vi "Stimulus-Initialize (V3).vi"(0 "Stimulus Channel":T1={"Waveform"={"Type"=enum."OFF", "Tone"={"Frequency (kHz)"=0.0, "Last Freq"=0.0, "Last Phase"=0.0}, "Pulse Train"={"Pulse width (us)"=0.0, "Pulse rate (Hz)"=0.0, "Gap (ms)"=0.0, "Polarity"=enum."POS", "PT State"={"Template"=[], "Nperiod"=0, "Index"=0, "Pulse Rate (Hz)"=0.0, "Phase (cycles)"=0.0, "Noff"=0}, "Asynch"=FALSE}, "Noise"={"InvFilt"=FALSE, "Noise"=[], "CurPt"=0, "Aweight"=FALSE, "Seed"=0, "afile"=path ""}, "File"={"Filename"=path "", "Signal"=[], "Channel"=0, "stream"=FALSE, "offset"=0, "nreps"=0, "loops"=0}, "FMSweep"={"Rate (oct/s)"=0.0, "Fmin (Hz)"=0.0, "Fmax (Hz)"=0.0, "Ramp (ms)"=0.0, "Linear"=FALSE}, "Chirp Train"={"Params"={"Fmin (kHz)"=4.0, "Fmax (kHz)"=64.0, "Compensate"=FALSE, "Duration (ms)"=2.0}, "Data"={"WF"=[]}}, "Complex Tone"={"Params"={"F0 (Hz)"=0.0, "Band"={"Flow (Hz)"=0.0, "Fhigh (Hz)"=0.0}, "Phase"=enum."Cosine", "Min F0 (Hz)"=0.0, "Max F0 (Hz)"=0.0, "ContinRandPhase"=FALSE, "Max peak factor"=inf, "Max mod depth"=2.0, "MinHarmNum"=0, "MaxHarmNum"=0, "Level Mode"=enum."per component", "% jitter"=0.0}, "Data"={"Ncomp"=0, "MinHarm"=0, "Phase"=[], "Amplitude"=[], "Npts/frame"=0, "Last F0"=0.0, "Fmin"=0.0, "Fmax"=0.0, "Lslope"=0.0, "randphase"=FALSE, "overall rms"=FALSE, "fmult"=[], "jittered"=FALSE}}, "Moving Ripple"={"Params"={"Fmin"=0.0, "Fmax"=0.0, "Density"=0.0, "Velocity"=0.0, "Depth"=0.0, "Phase"=0.0, "Comp/oct"=0}, "Data"={"Freq"=[], "A"=[], "phase"=[], "Phase"=0.0}}}, "Filter"={"Type"=enum."Lowpass", "CF (kHz)"=0.0, "BW (kHz)"=0.0, "Cascade"=FALSE, "Quadrature"=FALSE, "Scale Factor"=0.0, "Stages"=[], "Class"=enum."Elliptic", "Order"=0, "BWUnits"=enum."Linear"}, "Burst"={"Active"=FALSE, "Delay (ms)"=0.0, "Duration (ms)"=0.0, "Ramp (ms)"=0.0, "Rate (Hz)"=0.0, "Trepeat (ms)"=0.0, "Repeat"=FALSE}, "Level"={"Level"=0.0, "Units"=enum."dB atten", "Max"=0.0, "Multiplier"=0.0, "Cal File"=path "", "Cal"={"Freq (Hz)"=[], "Mag (dB SPL)"=[], "Phase (deg)"=[]}}, "Name"="", "Advanced"={"Rep Mask"="", "AltPol"=FALSE, "Var"="", "Expr"="", "Persist"=FALSE}, "SAM"={"Active"=FALSE, "Frequency (Hz)"=0.0, "Depth"=0.0, "Init Phase (cycles)"=0.0, "phase (degrees)"=0.0, "Asynch"=FALSE}, "Destination"={"Name"="", "Num"=0}} {"Filter"."Stages"."IIR Filter"."Forward Coefficients" format="%.4f"; "Filter"."Stages"."IIR Filter"."Reverse Coefficients" format="%.4f"}, 7 "Sampling rate (Hz)":dbl, 9 "Npts":i32, 11 "error in (no error)":errorcluster) -> (4 "Stimulus Channel out":T1={"Waveform"={"Type"=enum."OFF", "Tone"={"Frequency (kHz)"=0.0, "Last Freq"=0.0, "Last Phase"=0.0}, "Pulse Train"={"Pulse width (us)"=0.0, "Pulse rate (Hz)"=0.0, "Gap (ms)"=0.0, "Polarity"=enum."POS", "PT State"={"Template"=[], "Nperiod"=0, "Index"=0, "Pulse Rate (Hz)"=0.0, "Phase (cycles)"=0.0, "Noff"=0}, "Asynch"=FALSE}, "Noise"={"InvFilt"=FALSE, "Noise"=[], "CurPt"=0, "Aweight"=FALSE, "Seed"=0, "afile"=path ""}, "File"={"Filename"=path "", "Signal"=[], "Channel"=0, "stream"=FALSE, "offset"=0, "nreps"=0, "loops"=0}, "FMSweep"={"Rate (oct/s)"=0.0, "Fmin (Hz)"=0.0, "Fmax (Hz)"=0.0, "Ramp (ms)"=0.0, "Linear"=FALSE}, "Chirp Train"={"Params"={"Fmin (kHz)"=4.0, "Fmax (kHz)"=64.0, "Compensate"=FALSE, "Duration (ms)"=2.0}, "Data"={"WF"=[]}}, "Complex Tone"={"Params"={"F0 (Hz)"=0.0, "Band"={"Flow (Hz)"=0.0, "Fhigh (Hz)"=0.0}, "Phase"=enum."Cosine", "Min F0 (Hz)"=0.0, "Max F0 (Hz)"=0.0, "ContinRandPhase"=FALSE, "Max peak factor"=inf, "Max mod depth"=2.0, "MinHarmNum"=0, "MaxHarmNum"=0, "Level Mode"=enum."per component", "% jitter"=0.0}, "Data"={"Ncomp"=0, "MinHarm"=0, "Phase"=[], "Amplitude"=[], "Npts/frame"=0, "Last F0"=0.0, "Fmin"=0.0, "Fmax"=0.0, "Lslope"=0.0, "randphase"=FALSE, "overall rms"=FALSE, "fmult"=[], "jittered"=FALSE}}, "Moving Ripple"={"Params"={"Fmin"=0.0, "Fmax"=0.0, "Density"=0.0, "Velocity"=0.0, "Depth"=0.0, "Phase"=0.0, "Comp/oct"=0}, "Data"={"Freq"=[], "A"=[], "phase"=[], "Phase"=0.0}}}, "Filter"={"Type"=enum."Lowpass", "CF (kHz)"=0.0, "BW (kHz)"=0.0, "Cascade"=FALSE, "Quadrature"=FALSE, "Scale Factor"=0.0, "Stages"=[], "Class"=enum."Elliptic", "Order"=0, "BWUnits"=enum."Linear"}, "Burst"={"Active"=FALSE, "Delay (ms)"=0.0, "Duration (ms)"=0.0, "Ramp (ms)"=0.0, "Rate (Hz)"=0.0, "Trepeat (ms)"=0.0, "Repeat"=FALSE}, "Level"={"Level"=0.0, "Units"=enum."dB atten", "Max"=0.0, "Multiplier"=0.0, "Cal File"=path "", "Cal"={"Freq (Hz)"=[], "Mag (dB SPL)"=[], "Phase (deg)"=[]}}, "Name"="", "Advanced"={"Rep Mask"="", "AltPol"=FALSE, "Var"="", "Expr"="", "Persist"=FALSE}, "SAM"={"Active"=FALSE, "Frequency (Hz)"=0.0, "Depth"=0.0, "Init Phase (cycles)"=0.0, "phase (degrees)"=0.0, "Asynch"=FALSE}, "Destination"={"Name"="", "Num"=0}} {"Filter"."Stages"."IIR Filter"."Forward Coefficients" format="%.4f"; "Filter"."Stages"."IIR Filter"."Reverse Coefficients" format="%.4f"}, 6 "Max Level":dbl, 15 "error out":errorcluster)   [LabVIEW 2015]
uses:
  Controls/Advanced Filter XCtl/Filter Data.ctl
  Controls/Advanced Filter XCtl/Advanced Filter XCtl.xctl
  Controls/Level XCtl/Level Units.ctl
  Controls/Level XCtl/Level Data.ctl
  Controls/Level XCtl/Level XCtl.xctl
  Controls/Burst XCtl/Burst Data.ctl
  Controls/Burst XCtl/Burst Control.xctl
  Controls/Waveform XCtl/Waveform Enum.ctl
  Waveform VIs/Tone VIs/Tone Params.ctl
  Waveform VIs/Pulse Train VIs/Pulse Polarity.ctl
  Waveform VIs/Pulse Train VIs/PT-Continuous State.ctl
  Waveform VIs/Pulse Train VIs/Pulse Train Params.ctl
  Waveform VIs/Noise VIs/Noise Params.ctl
  Waveform VIs/File VIs/StimFile-Params.ctl
  Waveform VIs/FM Sweep VIs/FM Sweep Params.ctl
  Controls/Waveform XCtl/Waveform Data.ctl
  Controls/Waveform XCtl/Waveform XCtl.xctl
  Controls/Advanced Options XCtl/Advanced Stimulus Options.ctl
  Controls/Advanced Options XCtl/Advanced Stimulus Options.xctl
  Modulation VIs/SAM VIs/SAM Params.ctl
  Waveform VIs/Chirp Train VIs/Chirp Train Params.ctl
  Waveform VIs/Chirp Train VIs/Chirp Train.ctl
  Waveform VIs/Complex Tone VIs/CT-Phase Enum.ctl
  Waveform VIs/Complex Tone VIs/CT-Params.ctl
  Waveform VIs/Complex Tone VIs/CT-Runtime Data.ctl
  Filter VIs/Filter-Bandwidth Units.ctl
  V3 Controls/Typedefs/Destination.ctl
  V3 Controls/Stimulus Channel (V3)/Full Stimulus Channel Data.ctl
  Waveform VIs/Moving Ripple VIs/Moving Ripple.Params.ctl
  Waveform VIs/Moving Ripple VIs/Moving Ripple.Data.ctl
  Waveform VIs/Moving Ripple VIs/Moving Ripple.ctl
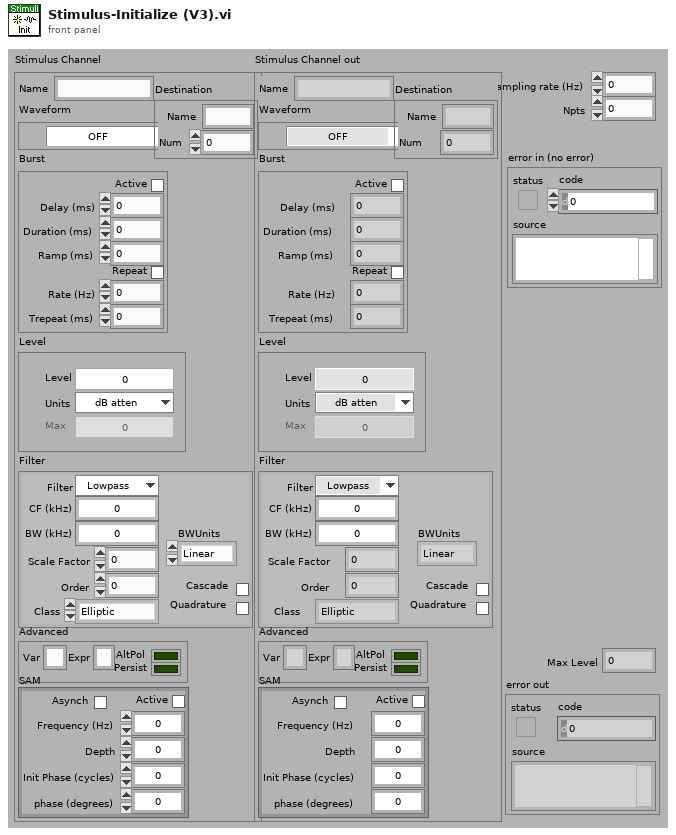
[diagram p1: front panel]
types:
  T1 = typedef "Stimulus Channel (V3).xctl/Full Stimulus Channel Data.ctl" = cluster{"Waveform":T2, "Filter":T19, "Burst":T21, "Level":T22, "Name":string, "Advanced":T24, "SAM":T25, "Destination":T26}
  T2 = typedef "Waveform XCtl.xctl/Waveform Data.ctl" = cluster{"Type":T3, "Tone":T4, "Pulse Train":T5, "Noise":T8, "File":T9, "FMSweep":T10, "Chirp Train":T11, "Complex Tone":cluster{"Params":T13, "Data":T15}, "Moving Ripple":T16}
  T3 = typedef "Waveform Enum.ctl" = enum16{"OFF", "Tone", "Noise", "Pulse Train", "File", "FM Sweep", "Chirp Train", "Complex Tone", "FM Tone", "Moving Ripple"}
  T4 = typedef "Tone Params.ctl" = cluster{"Frequency (kHz)":dbl, "Last Freq":dbl, "Last Phase":dbl}
  T5 = typedef "Pulse Train Params.ctl" = cluster{"Pulse width (us)":dbl, "Pulse rate (Hz)":dbl, "Gap (ms)":dbl, "Polarity":T6, "PT State":T7, "Asynch":bool}
  T6 = typedef "Pulse Polarity.ctl" = enum16{"POS", "NEG", "POS-NEG", "NEG-POS"}
  T7 = typedef "PT-Continuous State.ctl" = cluster{"Template":dbl[], "Nperiod":i32, "Index":i32, "Pulse Rate (Hz)":dbl, "Phase (cycles)":dbl, "Noff":i32}
  T8 = typedef "Noise Params.ctl" = cluster{"InvFilt":bool, "Noise":dbl[], "CurPt":i32, "Aweight":bool, "Seed":i32, "afile":path}
  T9 = typedef "StimFile-Params.ctl" = cluster{"Filename":path, "Signal":dbl[], "Channel":i32, "stream":bool, "offset":i32, "nreps":i32, "loops":i32}
  T10 = typedef "FM Sweep Params.ctl" = cluster{"Rate (oct/s)":dbl, "Fmin (Hz)":dbl, "Fmax (Hz)":dbl, "Ramp (ms)":dbl, "Linear":bool}
  T11 = typedef "Chirp Train.ctl" = cluster{"Params":T12, "Data":cluster{"WF":dbl[]}}
  T12 = typedef "Chirp Train Params.ctl" = cluster{"Fmin (kHz)":dbl, "Fmax (kHz)":dbl, "Compensate":bool, "Duration (ms)":dbl}
  T13 = typedef "CT-Params.ctl" = cluster{"F0 (Hz)":dbl, "Band":cluster{"Flow (Hz)":dbl, "Fhigh (Hz)":dbl}, "Phase":T14, "Min F0 (Hz)":dbl, "Max F0 (Hz)":dbl, "ContinRandPhase":bool, "Max peak factor":dbl, "Max mod depth":dbl, "MinHarmNum":i32, "MaxHarmNum":i32, "Level Mode":enum16{"per component", "overall rms"}, "% jitter":dbl}
  T14 = typedef "CT-Phase Enum.ctl" = enum16{"Cosine", "Random", "Alternating"}
  T15 = typedef "CT-Runtime Data.ctl" = cluster{"Ncomp":i32, "MinHarm":i32, "Phase":dbl[], "Amplitude":dbl[], "Npts/frame":i32, "Last F0":dbl, "Fmin":dbl, "Fmax":dbl, "Lslope":dbl, "randphase":bool, "overall rms":bool, "fmult":dbl[], "jittered":bool}
  T16 = typedef "Moving Ripple.ctl" = cluster{"Params":T17, "Data":T18}
  T17 = typedef "Moving Ripple.Params.ctl" = cluster{"Fmin":dbl, "Fmax":dbl, "Density":dbl, "Velocity":dbl, "Depth":dbl, "Phase":dbl, "Comp/oct":i32}
  T18 = typedef "Moving Ripple.Data.ctl" = cluster{"Freq":dbl[], "A":dbl[], "phase":dbl[], "Phase":dbl}
  T19 = typedef "Advanced Filter XCtl.xctl/Filter Data.ctl" = cluster{"Type":enum16{"Lowpass", "Highpass", "Bandpass", "Bandstop", "OFF"}, "CF (kHz)":dbl, "BW (kHz)":dbl, "Cascade":bool, "Quadrature":bool, "Scale Factor":dbl, "Stages":cluster{"IIR Filter":cluster{"filter structure":enum32{"IIR 2nd Order", "IIR 4th Order"}, "Reverse Coefficients":dbl[], "Forward Coefficients":dbl[]}, "State":dbl[]}[], "Class":enum16{"Elliptic", "Butterworth"}, "Order":i32, "BWUnits":T20}
  T20 = typedef "Filter-Bandwidth Units.ctl" = enum16{"Linear", "Octaves", "Min-Max"}
  T21 = typedef "Burst Control.xctl/Burst Data.ctl" = cluster{"Active":bool, "Delay (ms)":dbl, "Duration (ms)":dbl, "Ramp (ms)":dbl, "Rate (Hz)":dbl, "Trepeat (ms)":dbl, "Repeat":bool}
  T22 = typedef "Level XCtl.xctl/Level Data.ctl" = cluster{"Level":dbl, "Units":T23, "Max":dbl, "Multiplier":dbl, "Cal File":path, "Cal":cluster{"Freq (Hz)":dbl[], "Mag (dB SPL)":dbl[], "Phase (deg)":dbl[]}}
  T23 = typedef "Level Units.ctl" = enum16{"dB atten", "dB SPL", "dB re 1 Vrms", "dB V/Hz½", "mW", "dB HL", "Volts", "dB mW"}
  T24 = typedef "Advanced Stimulus Options.xctl/Advanced Stimulus Options.ctl" = cluster{"Rep Mask":string, "AltPol":bool, "Var":string, "Expr":string, "Persist":bool}
  T25 = typedef "SAM Params.ctl" = cluster{"Active":bool, "Frequency (Hz)":dbl, "Depth":dbl, "Init Phase (cycles)":dbl, "phase (degrees)":dbl, "Asynch":bool}
  T26 = typedef "Destination.ctl" = cluster{"Name":string, "Num":i32}
  T27 = enum16{"Lowpass", "Highpass", "Bandpass", "Bandstop", "OFF"}
  T28 = enum16{"Clear", "Set data", "Reset index", "Get data"}
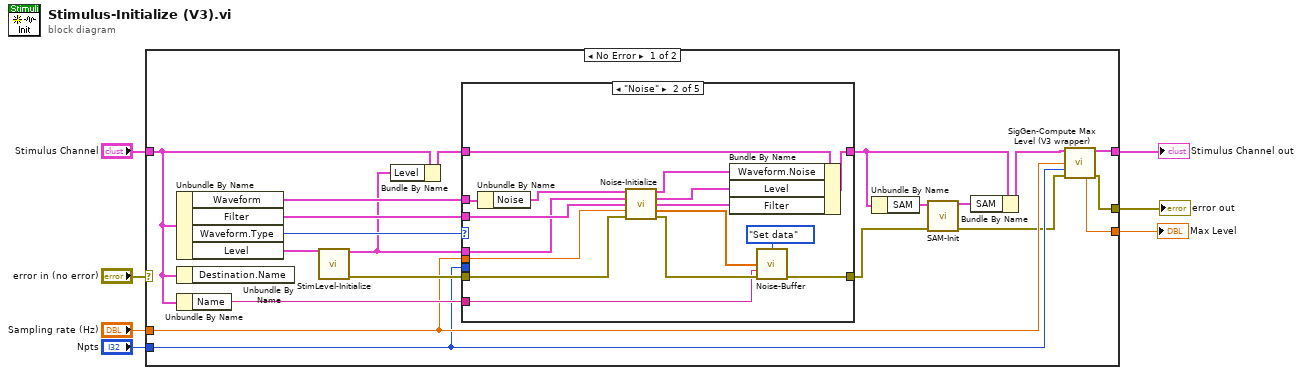
[diagram p0: block diagram]
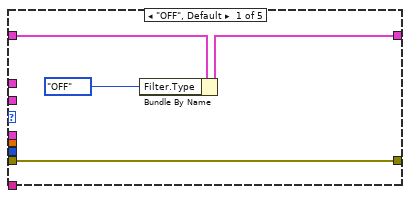
[diagram p2: hidden frame]
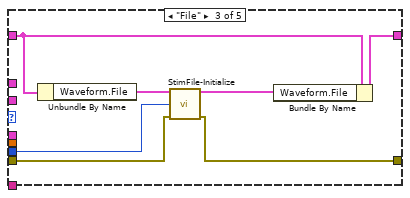
[diagram p3: hidden frame]
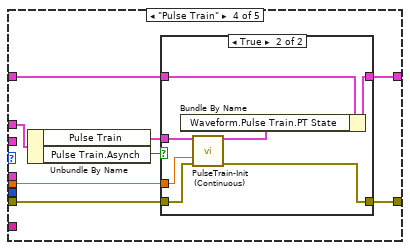
[diagram p4: hidden frame]
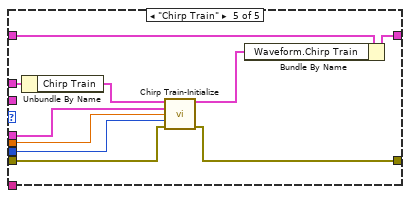
[diagram p6: hidden frame]
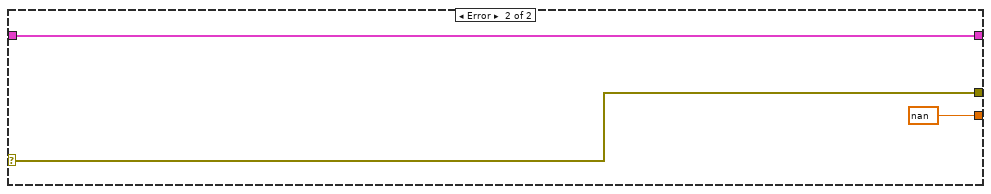
[diagram p7: hidden frame]
diagram:
  n1 = case shown="No Error" "error in (no error)" {
    selector: "error in (no error)" -> [_ w84]
    tunnel: "Sampling rate (Hz)" -> [w13 _]
    tunnel: [w15 w83] -> w3
    tunnel: [w9 w84] -> w5
    tunnel: "Stimulus Channel" -> [w8 w83]
    tunnel: "Npts" -> [w12 _]
    tunnel: [w10 nan ("Max Level")] -> w1
    frame No Error {
      n2 = Unbundle By Name(w8) -> ("Waveform"=w25:T2, "Filter"=w26:T19, "Waveform.Type"=w27:T3, "Level"=w19:T22)
      n3 = Unbundle By Name(w8) -> ()  [unwired: 1 out]
      n4 = Unbundle By Name(w8) -> ("Name"=w16:string)
      n5 = call "StimLevel-Initialize.vi"("Level"=w19) -> ("Level out"=w17:T22, "error out"=w20:errorcluster)  [unwired: 13 in]
      n6 = Bundle By Name(cluster=w8, "Level"=w17) -> (w18:T1)
      n7 = case shown="\"Noise\"" w27 {
        tunnel: w26 -> [_ w45 _ _ _]
        tunnel: w13 -> [_ w47 _ w55 w74]
        tunnel: w20 -> [w31 w46 w50 w57 w78]
        tunnel: w18 -> [w30 w33 w54 w60 w81]
        tunnel: [w29 w41 w53 w59 w79] -> w24
        tunnel: [w31 w36 w49 w56 w77] -> w22
        tunnel: w12 -> [_ _ w48 _ w73]
        tunnel: w25 -> [_ w43 _ w62 w80]
        tunnel: w17 -> [_ w44 _ _ w72]
        tunnel: w16 -> [_ w32 _ _ _]
        frame "OFF", Default {
          n8 = Bundle By Name(cluster=w30, "Filter.Type"=T27."OFF") -> (w29:T1)
        }
        frame "Noise" {
          n9 = Unbundle By Name(w43) -> ("Noise"=w42:T8)
          n10 = call "Noise-Initialize.vi"("Noise"=w42, "Level"=w44, "Filter"=w45, "Sampling rate (Hz)"=w47, "error in (no error)"=w46) -> ("Noise Out"=w40:T8, "Level Out"=w39:T22, "Filter Out"=w38:T19, "Noise"=w34:dbl[], "error out"=w37:errorcluster)  [unwired: 6 in]
          n11 = Bundle By Name(cluster=w33, "Waveform.Noise"=w40, "Level"=w39, "Filter"=w38) -> (w41:T1)
          n12 = call "Noise-Buffer.vi"("Action"=T28."Set data", "Data In"=w34, "Name"=w32, "error in (no error)"=w37) -> ("error out"=w36:errorcluster)  [unwired: 10 in, 1 out]
        }
        frame "File" {
          n13 = Unbundle By Name(w54) -> ("Waveform.File"=w52:T9)
          n14 = call "StimFile-Initialize.vi"("File"=w52, "Npts"=w48, "error in (no error)"=w50) -> ("File out"=w51:T9, "error out"=w49:errorcluster)  [unwired: 11 in]
          n15 = Bundle By Name(cluster=w54, "Waveform.File"=w51) -> (w53:T1)
        }
        frame "Pulse Train" {
          n16 = Unbundle By Name(w62) -> ("Pulse Train"=w58:T5, "Pulse Train.Asynch"=w61:bool)
          n17 = case shown="True" w61 {
            tunnel: w60 -> [w64 w67]
            tunnel: [w64 w66] -> w59
            tunnel: w58 -> [_ w71]
            tunnel: w57 -> [w63 w70]
            tunnel: [w63 w69] -> w56
            tunnel: w55 -> [_ w68]
            frame False {
            }
            frame True {
              n18 = call "PulseTrain-Init (Continuous).vi"("Pulse Train Params"=w71, "Fs (Hz)"=w68, "error in (no error)"=w70) -> ("Initial State"=w65:T7, "error out"=w69:errorcluster)  [unwired: 11 in]
              n19 = Bundle By Name(cluster=w67, "Waveform.Pulse Train.PT State"=w65) -> (w66:T1)
            }
          }
        }
        frame "Chirp Train" {
          n20 = Unbundle By Name(w80) -> ("Chirp Train"=w76:T11)
          n21 = call "Chirp Train-Initialize.vi"("Chirp Train in"=w76, "Level"=w72, "Sampling rate (Hz)"=w74, "Npts"=w73, "error in (no error)"=w78) -> ("Chirp Train out"=w75:T11, "error out"=w77:errorcluster)  [unwired: 9 in]
          n22 = Bundle By Name(cluster=w81, "Waveform.Chirp Train"=w75) -> (w79:T1)
        }
      }
      n23 = Unbundle By Name(w24) -> ("SAM"=w23:T25)
      n24 = call "SAM-Init.vi"("SAM In"=w23, "error in (no error)"=w22) -> ("SAM Out"=w21:T25, "error out"=w11:errorcluster)  [unwired: 12 in]
      n25 = Bundle By Name(cluster=w24, "SAM"=w21) -> (w14:T1)
      n26 = call "SigGen-Compute Max Level (V3 wrapper).vi"("Stimulus Channel"=w14, "Sampling Rate (Hz)"=w13, "Npts"=w12, "error in (no error)"=w11) -> ("Stimulus Channel out"=w15:T1, "Max Level"=w10:dbl, "error out"=w9:errorcluster)  [unwired: 9 in]
    }
    frame Error {
    }
  }
  "error out" <- w5
  "Stimulus Channel out" <- w3
  "Max Level" <- w1
